vi "Process_Commands.vi"(10 "All_Sensor_Readings":T4, 11 "All Driver Commands":T1) -> (3 "All_Outputs":T8)   [LabVIEW 2012]
uses:
  All_Outputs.ctl
  Cirular Shooter/Shooter_Outputs.ctl
  Climber/Climber_Outputs.ctl
  All_Sensor_Readings.ctl
  Climber/climber_sensor_readings.ctl
  Cirular Shooter/Shooter_inputs.ctl
  Field Drive/Field_Drive_out.ctl
  All_Commands.ctl
  Cirular Shooter/circular_shooter_commands.ctl
  Climber/Climber_Commands.ctl
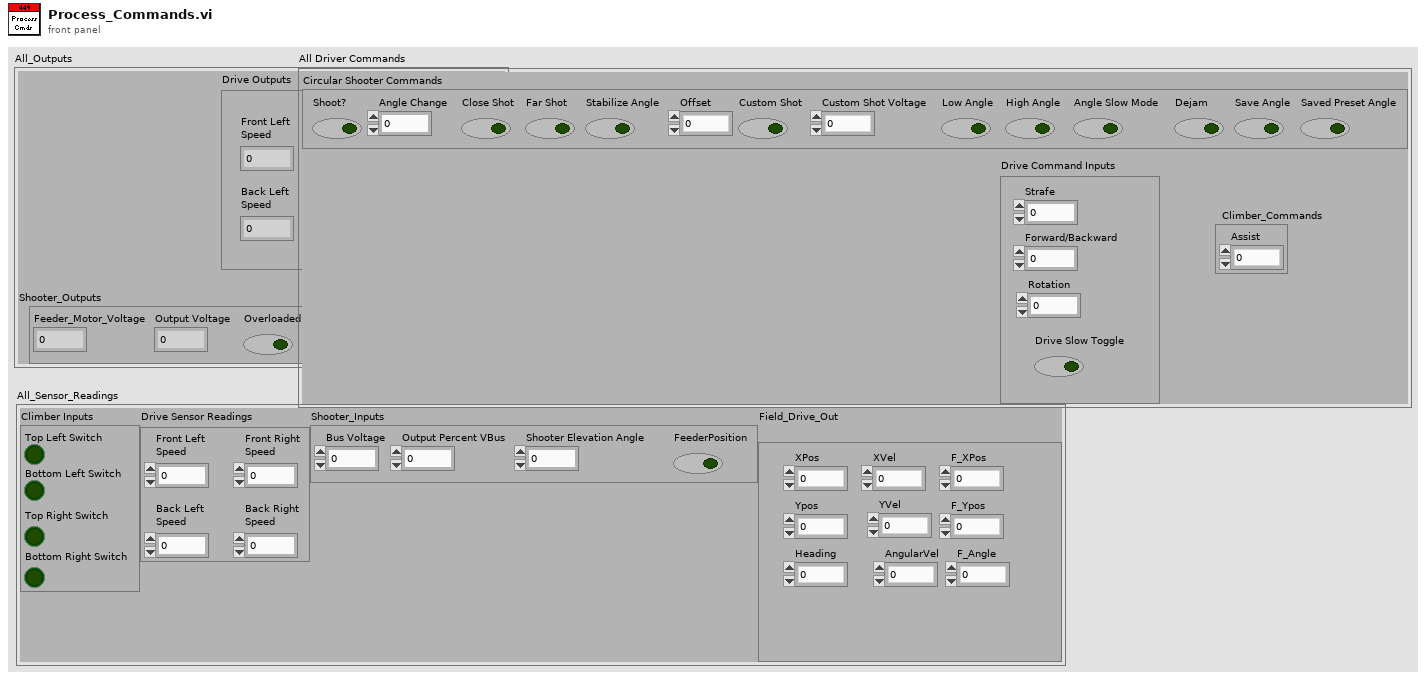
[diagram p1: front panel]
types:
  T1 = typedef "All_Commands.ctl" = cluster{"Circular Shooter Commands":T2, "Drive Command Inputs":cluster{"Strafe":dbl, "Forward/Backward":dbl, "Rotation":dbl, "Drive Slow Toggle":bool}, "Climber_Commands":T3}
  T2 = typedef "circular_shooter_commands.ctl" = cluster{"Shoot?":bool, "Angle Change":dbl, "Close Shot":bool, "Far Shot":bool, "Stabilize Angle ":bool, "Offset":dbl, "Custom Shot":bool, "Custom Shot Voltage":dbl, "Low Angle":bool, "High Angle":bool, "Angle Slow Mode":bool, "Dejam":bool, "Save Angle":bool, "Saved Preset Angle":bool}
  T3 = typedef "Climber_Commands.ctl" = cluster{"Assist":dbl}
  T4 = typedef "All_Sensor_Readings.ctl" = cluster{"Climber Inputs":T5, "Drive Sensor Readings":cluster{"Front Left\nSpeed":dbl, "Back Left\nSpeed":dbl, "Front Right\nSpeed":dbl, "Back Right\nSpeed":dbl}, "Shooter_Inputs":T6, "Field_Drive_Out\n":T7}
  T5 = typedef "climber_sensor_readings.ctl" = cluster{"Top Left Switch":bool, "Bottom Left Switch":bool, "Top Right Switch":bool, "Bottom Right Switch":bool}
  T6 = typedef "Shooter_inputs.ctl" = cluster{"Bus Voltage":dbl, "Output Percent VBus":dbl, "Shooter Elevation Angle":dbl, "FeederPosition":bool}
  T7 = typedef "Field_Drive_out.ctl" = cluster{"XPos":dbl, "Ypos":dbl, "XVel":dbl, "YVel":dbl, "Heading":dbl, "AngularVel":dbl, "F_XPos":dbl, "F_Ypos":dbl, "F_Angle":dbl}
  T8 = typedef "All_Outputs.ctl" = cluster{"Drive Outputs":cluster{"Front Left\nSpeed":dbl, "Back Left\nSpeed":dbl, "Front Right\nSpeed":dbl, "Back Right\nSpeed":dbl}, "Shooter_Outputs":T9, "Climber_Outputs":T10}
  T9 = typedef "Shooter_Outputs.ctl" = cluster{"Feeder_Motor_Voltage":dbl, "Output Voltage":dbl, "Overloaded":bool, "Variable_Angle_Voltage":dbl, "Saved Angle":dbl}
  T10 = typedef "Climber_Outputs.ctl" = cluster{"Assist Voltage":dbl}
  T11 = cluster{"Strafe":dbl, "Forward/Backward":dbl, "Rotation":dbl, "Drive Slow Toggle":bool}
  T12 = cluster{"Front Left\nSpeed":dbl, "Back Left\nSpeed":dbl, "Front Right\nSpeed":dbl, "Back Right\nSpeed":dbl}
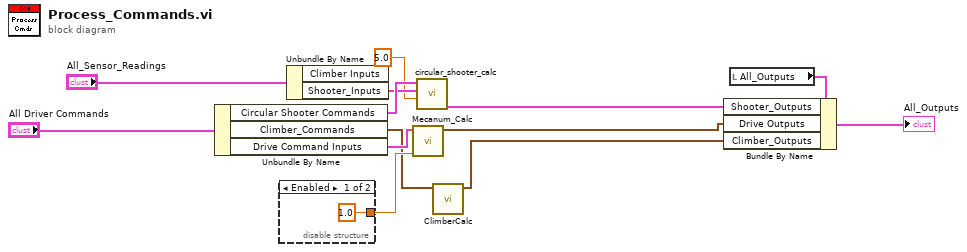
[diagram p0: block diagram]
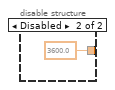
[diagram p2: hidden frame]
diagram:
  n1 = Unbundle By Name("All Driver Commands") -> ("Circular Shooter Commands"=w13:T2, "Climber_Commands"=w2:T3, "Drive Command Inputs"=w4:T11)
  n2 = disable-structure shown="Enabled" {
    disable-tunnel: [1.0 ("Max Speed") 3600.0 ("Max Speed")] -> w7
    frame Enabled {
    }
    frame Disabled {
    }
  }
  n3 = Unbundle By Name("All_Sensor_Readings") -> ("Shooter_Inputs"=w6:T6)  [unwired: 1 out]
  n4 = call "Mecanum_Calc.vi"("Max Speed"=w7, "Drive Command Inputs"=w4) -> ("Drive Outputs"=w12:T12)  [unwired: 8 in, 1 out]
  n5 = call "circular_shooter_calc.vi"("Shooting Speed"=5.0, "Shooter_Inputs"=w6, "Circular Shooter Commands"=w13) -> ("Shooter_Outputs"=w11:T9)  [unwired: 8 in]
  n6 = call "ClimberCalc.vi"("Climber_Commands"=w2) -> ("Climber_Outputs"=w1:T10)  [unwired: 9 in]
  n7 = local read "All_Outputs"() -> (w10:T8)
  n8 = Bundle By Name(cluster=w10, "Shooter_Outputs"=w11, "Drive Outputs"=w12, "Climber_Outputs"=w1) -> (→"All_Outputs":T8)
